vi "Multi Channel PID.vi"() -> ()   [LabVIEW 2023]
doc: "This example demonstrates how to create a independent PID controller for each input and output of the plant. If plant has interconnections between channels, use decoupler before calling the PID function."
uses:
  <vilib>/addons/control/pid/pid.llb/PID (DBL Array).vi
  <vilib>/addons/control/pid/NI_PID_pid.lvlib
panel:
  in  "Loop":i32=1 min=1 max=5
  in  "derivative time (Td, min)":dbl format="%.3f"
  in  "integral time (Ti, min)":dbl=0.1 format="%.3f"
  in  "proportional gain (Kc)":dbl=40.0 format="%.3f"
  in  "SP:":dbl(slide)=10.119047619047619 min=0.0 max=0.0 scale=0.0..100.0
  out "MV:":dbl(slide)=17.27086786797185 scale=-100.0..100.0
  out "PV:":dbl(slide)=9.982717347355862 scale=0.0..100.0
  in  "Loop 5":cluster{dbl, dbl}(slide)={33.333333333333336, 33.17061230277219} scale=0.0..100.0
  in  "Loop 4":cluster{dbl, dbl}(slide)={73.21428571428571, 72.91679954674115} scale=0.0..100.0
  in  "Loop 3":cluster{dbl, dbl}(slide)={16.666666666666668, 16.537798468500863} scale=0.0..100.0
  in  "Loop 2":cluster{dbl, dbl}(slide)={54.13533834586466, 53.967433610574744} scale=0.0..100.0
  in  "Loop 1":cluster{dbl, dbl}(slide)={10.119047619047619, 9.982717347355862} scale=0.0..100.0
  in  "Load 5":dbl(slide)=58.0 scale=0.0..100.0
  in  "Load 4":dbl(slide)=58.0 scale=0.0..100.0
  in  "Load 3":dbl(slide)=58.0 scale=0.0..100.0
  in  "Load 2":dbl(slide)=58.0 scale=0.0..100.0
  in  "Gain 5":dbl(slide)=2.642857142857143 scale=0.0..5.0
  in  "Gain 3":dbl(slide)=3.2203389830508473 scale=0.0..5.0
  in  "Gain 4":dbl(slide)=2.642857142857143 scale=0.0..5.0
  in  "Load 1":dbl(slide)=58.0 scale=0.0..100.0
  in  "Gain 1":dbl(slide)=3.2203389830508473 scale=0.0..5.0
  in  "Gain 2":dbl(slide)=2.642857142857143 scale=0.0..5.0
  in  "Stop":bool
  out "Process Variable and Setpoint":T1(graph)={10.119047619047619, 54.13533834586466, 16.666666666666668, 73.21428571428571, 33.333333333333336, "initial PV"=9.982717347355862, "initial PV"=53.967433610574744, "initial PV"=16.537798468500863, "initial PV"=72.91679954674115, "initial PV"=33.17061230277219}
  # "Overview: This example demonstrates how to create a independent PID controller for each input and output of the plant. If plant has interconnections between channels, use decoupler before calling the PID function.\nInstructions:\n1. Run the VI.\n2. Choose the Loop you want to control. The PID parameters will be change only for that Loop.\n3. Click Stop to stop the VI."
  # "PID Parameters"
  # "Plants Parameters"
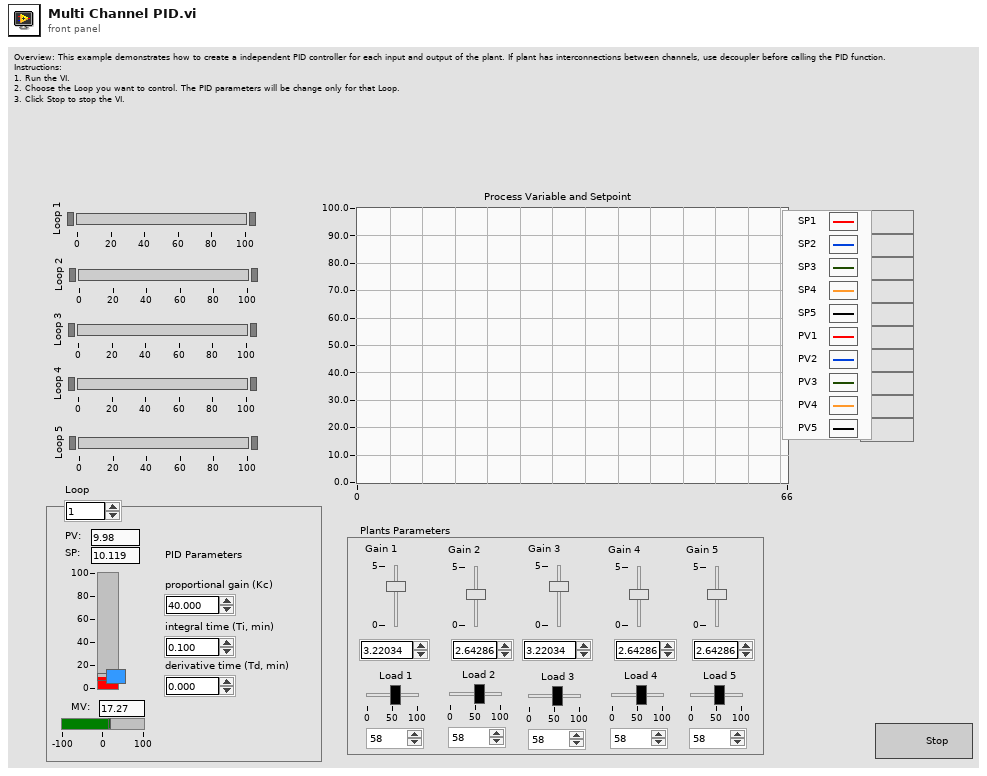
[diagram p1: front panel]
types:
  T1 = cluster{dbl, dbl, dbl, dbl, dbl, "initial PV":dbl, "initial PV":dbl, "initial PV":dbl, "initial PV":dbl, "initial PV":dbl}
  T2 = cluster{"proportional gain (Kc)":dbl, "integral time (Ti, min)":dbl, "derivative time (Td, min)":dbl}
  T3 = cluster{"proportional gain (Kc)":dbl, "integral time (Ti, min)":dbl, "derivative time (Td, min)":dbl}[]
  T4 = cluster{"static gain":dbl, "lag (min)":dbl, "dead cycles":i32, "load %":dbl, "deadband":dbl, "noise level %":dbl, "initial PV":dbl}
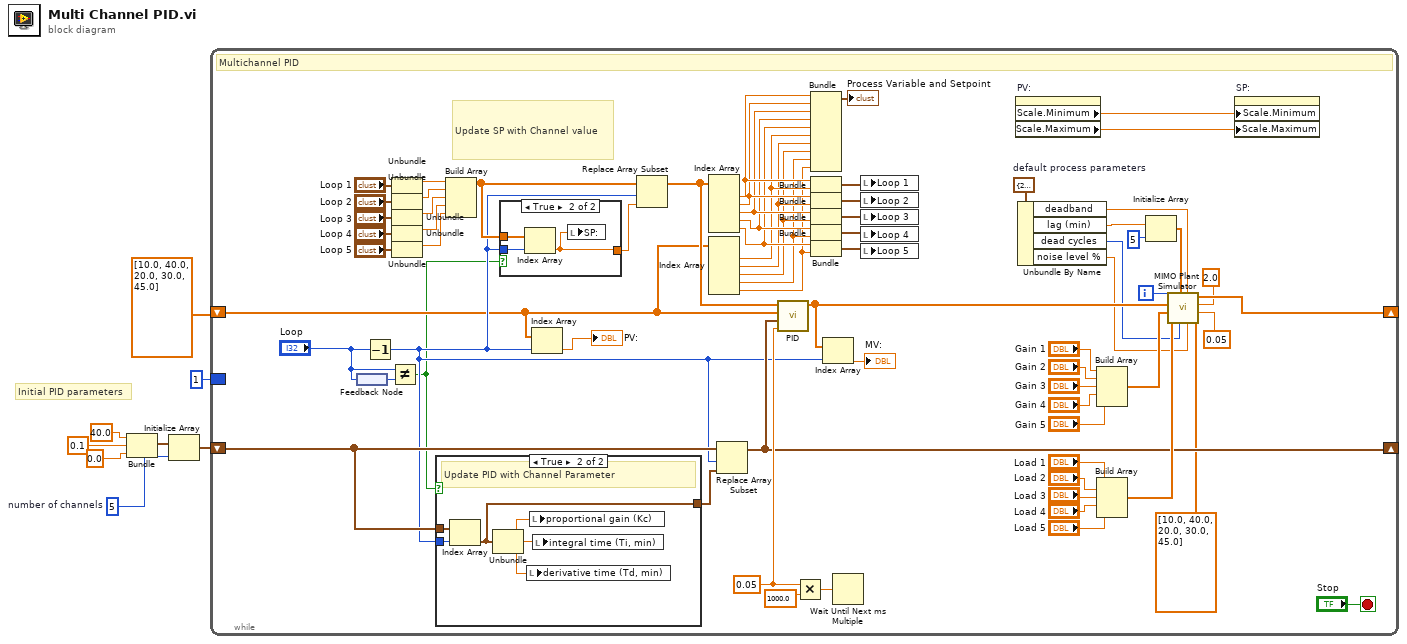
[diagram p0: block diagram]
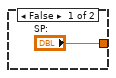
[diagram p2: hidden frame]
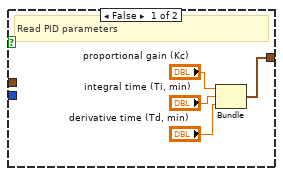
[diagram p3: hidden frame]
diagram:
  w6 = 5  # number of channels
  # "Initial PID parameters"
  n1 = Bundle("proportional gain (Kc)"=40.0, "integral time (Ti, min)"=0.1, "derivative time (Td, min)"=0.0) -> (w7:T2)  [unwired: 1 in]
  n2 = Initialize Array(w7, w6) -> (w5:T3)
  n3 = while {
    shift-left: dbl[] [10.0, 40.0, 20.0, 30.0, 45.0] -> [w37]
    shift-right: [w75] -> _
    shift-right: [w42] -> _
    shift-left: w5 -> [w41]
    border: 1 ("Loop") -> [_]
    i -> [w76]
    stop <- "Stop" stop-if-true
    w18 = T4 {"static gain"=2.5, "lag (min)"=0.5, "dead cycles"=0, "load %"=40.0, "deadband"=2.0, "noise level %"=50.0, "initial PV"=0.0}  # default process parameters
    w72 = 0.05 ("Sampling Time dt (s)")
    # "Update SP with Channel value"
    # "Multichannel PID"
    n4 = feedback-in #1("Loop") -> ()
    n5 = feedback #1() -> (w33:i32)
    n6 = Decrement(x="Loop") -> (x-1=w39:i32)
    n7 = Not Equal?(x="Loop", y=w33) -> (x != y?=w35:bool)
    n8 = Unbundle("Loop 1") -> (w55:dbl)  [unwired: 1 out]
    n9 = Unbundle("Loop 2") -> (w49:dbl)  [unwired: 1 out]
    n10 = Unbundle("Loop 3") -> (w36:dbl)  [unwired: 1 out]
    n11 = Unbundle("Loop 4") -> (w48:dbl)  [unwired: 1 out]
    n12 = Unbundle("Loop 5") -> (w47:dbl)  [unwired: 1 out]
    n13 = case shown="True" w35 {
      tunnel: [w83 w88] -> w43
      tunnel: w41 -> [_ w92]
      tunnel: w39 -> [_ w87]
      frame False {
        # "Read PID parameters"
        n14 = Bundle("proportional gain (Kc)"="proportional gain (Kc)", "integral time (Ti, min)"="integral time (Ti, min)", "derivative time (Td, min)"="derivative time (Td, min)") -> (w83:T2)  [unwired: 1 in]
      }
      frame True {
        # "Update PID with Channel Parameter"
        n15 = Index Array(array=w92, index=w87) -> (element=w88:T2)
        n16 = Unbundle(w88) -> ("proportional gain (Kc)"=w91:dbl, "integral time (Ti, min)"=w90:dbl, "derivative time (Td, min)"=w89:dbl)
        n17 = local write "derivative time (Td, min)"(w89) -> ()
        n18 = local write "proportional gain (Kc)"(w91) -> ()
        n19 = local write "integral time (Ti, min)"(w90) -> ()
      }
    }
    n20 = Build Array(w55, w49, w36, w48, w47) -> (w40:dbl[])
    n21 = case shown="True" w35 {
      tunnel: w40 -> [_ w82]
      tunnel: w39 -> [_ w81]
      tunnel: ["SP:" w80] -> w38
      frame False {
      }
      frame True {
        n22 = Index Array(array=w82, index=w81) -> (element=w80:dbl)
        n23 = local write "SP:"(w80) -> ()
      }
    }
    n24 = Index Array(array=w37, index=w39) -> (element=→"PV:":dbl)
    n25 = Replace Array Subset(array=w40, new element=w38, index=w39) -> (w44:dbl[])
    n26 = Index Array(array=w44) -> (element #1=w32:dbl, element #2=w31:dbl, element #3=w30:dbl, element #4=w29:dbl, element #5=w28:dbl)  [unwired: 5 in]
    n27 = Index Array(array=w37) -> (element #1=w27:dbl, element #2=w26:dbl, element #3=w25:dbl, element #4=w24:dbl, element #5=w23:dbl)  [unwired: 5 in]
    n28 = Replace Array Subset(array=w41, new element=w43, index=w39) -> (w42:T3)
    n29 = call-poly <vilib>:"PID.vi"("dt (s)"=w72, "PID gains"=w42, "process variable"=w37, "setpoint"=w44) -> ("output"=w45:dbl[])  [unwired: 6 in, 1 out]
    n30 = Multiply(x=w72, y=1000.0) -> (x*y=w20:dbl)
    n31 = Bundle(w32, w31, w30, w29, w28, "initial PV"=w27, "initial PV"=w26, "initial PV"=w25, "initial PV"=w24, "initial PV"=w23) -> (→"Process Variable and Setpoint":T1)  [unwired: 1 in]
    n32 = Bundle(w32, "initial PV"=w27) -> (w54:cluster{dbl, "initial PV":dbl})  [unwired: 1 in]
    n33 = Bundle(w31, "initial PV"=w26) -> (w53:cluster{dbl, "initial PV":dbl})  [unwired: 1 in]
    n34 = Bundle(w30, "initial PV"=w25) -> (w52:cluster{dbl, "initial PV":dbl})  [unwired: 1 in]
    n35 = Bundle(w29, "initial PV"=w24) -> (w51:cluster{dbl, "initial PV":dbl})  [unwired: 1 in]
    n36 = Bundle(w28, "initial PV"=w23) -> (w50:cluster{dbl, "initial PV":dbl})  [unwired: 1 in]
    n37 = Index Array(array=w45, index=w39) -> (element=→"MV:":dbl)
    n38 = Wait Until Next ms Multiple(millisecond multiple=w20) -> ()  [unwired: 1 out]
    n39 = local write "Loop 1"(w54) -> ()
    n40 = local write "Loop 2"(w53) -> ()
    n41 = local write "Loop 3"(w52) -> ()
    n42 = local write "Loop 4"(w51) -> ()
    n43 = local write "Loop 5"(w50) -> ()
    n44 = property on="PV:" class="Slide (strict)"() -> ("Scale.Minimum"=w74:dbl, "Scale.Maximum"=w73:dbl)  [unwired: 2 in, 2 out]
    n45 = Unbundle By Name(w18) -> ("deadband"=w15:dbl, "lag (min)"=w17:dbl, "dead cycles"=w13:i32, "noise level %"=w12:dbl)
    n46 = Build Array("Gain 1", "Gain 2", "Gain 3", "Gain 4", "Gain 5") -> (w67:dbl[])
    n47 = Build Array("Load 1", "Load 2", "Load 3", "Load 4", "Load 5") -> (w61:dbl[])
    n48 = Initialize Array(w17, 5) -> (w14:dbl[])
    n49 = call "MIMO Plant Simulator.vi"("Initial PV"=dbl[] [10.0, 40.0, 20.0, 30.0, 45.0], "dt (s)"=0.05 ("Sampling Time dt (s)"), "Measurement Noise (%)"=2.0, "Controller Noise (%)"=w12, "Valve Deadband"=w15, "Process Deadtime"=w13, "Lags"=w14, "Plant Load"=w61, "Plant Gains"=w67, "Manipulated Variable (MV)"=w45, "iteration"=w76) -> ("Process Variable"=w75:dbl[])
    n50 = property on="SP:" class="Slide (strict)"("Scale.Minimum"=w74, "Scale.Maximum"=w73) -> ()  [unwired: 2 in, 2 out]
  }
